vi "Create File.vi"(8 "error in (no error)":errorcluster, 10 "operation (replace)":T1(ring)=enum."replace or create", 11 "Path":path) -> (0 "error out":errorcluster, 3 "TIFF Writer out":refnum<class "TIFF Writer.lvclass">)   [LabVIEW 2020, in "LV Tiff.lvlib" / "TIFF Writer.lvclass"]
uses:
  TIFF Writer.lvclass
  TIFF Writer.lvclass/TIFF Writer.ctl
  LV Tiff.lvlib
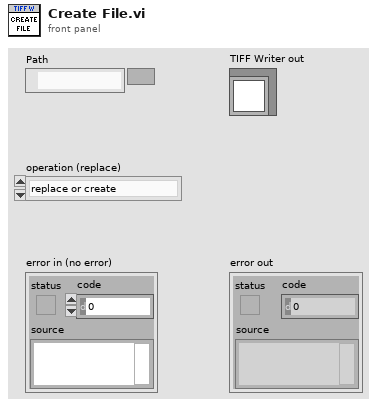
[diagram p1: front panel]
types:
  T1 = enum16{"open", "replace", "create", "open or create", "replace or create", "replace or create with confirmation"}
  T2 = enum16{"big-endian, network order", "native, host order", "little-endian"}
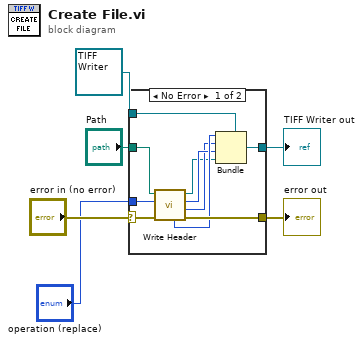
[diagram p0: block diagram]
diagram:
  n1 = case shown="No Error" "error in (no error)" {
    selector: "error in (no error)" -> [w14 w18]
    tunnel: [w13 w18] -> w5
    tunnel: [w12 w17] -> w3
    tunnel: refnum<class "TIFF Writer.lvclass"> refnum ("TIFF Writer in") -> [w16 w17]
    tunnel: "Path" -> [w15 _]
    tunnel: "operation (replace)" -> [w7 _]
    frame No Error {
      n2 = call "Write Header.vi"("error in (no error)"=w14, "operation (replace)"=w7, "Path"=w15) -> ("error out"=w13:errorcluster, "IFD Offset Position"=w9:i64, "Offset"=w10:i32, "Byte Stream File out"=w8:refnum<file>, "byte order (0:big-endian, network order)"=w11:T2)  [unwired: 4 in]
      n3 = Bundle(cluster=w16, w11, w9, w10, w8) -> (w12:refnum<class "TIFF Writer.lvclass">)
    }
    frame Error {
    }
  }
  "error out" <- w5
  "TIFF Writer out" <- w3
